vi "main.vi"() -> ()   [LabVIEW 2020]
uses:
  Function/TypeDef/TestFlow.ctl
  <vilib>/Utility/file.llb/Read From Spreadsheet File (string).vi
  <vilib>/Utility/file.llb/Write Delimited Spreadsheet (string).vi
  <vilib>/Utility/file.llb/Read Delimited Spreadsheet (string).vi
panel:
  out "Counter":cluster{"第n筆":u32, "第N輪":u32, "經過時間(ms)":u32}={"第n筆"=1, "第N輪"=1, "經過時間(ms)"=0}
  in  "Test Condition":T1={"每一輪取n筆"=1, "每一輪間隔t時間(sec)"=30.0, "總共取N輪"=1, "開始自動測試"=FALSE} {"總共取N輪" min=1 max=10000; "每一輪間隔t時間(sec)" min=0.01 max=30000.0 format="%_3g"; "每一輪取n筆" min=1 max=10000}
  out "SPR efficiency":dbl
  out "SPR wavelength(nm)":dbl
  in  "結束測試":bool
  in  "OSA Setting":T2={"CENTER(nm)"="850", "SPAN(nm)"="700", "RESOLUTION(nm)"="10", "SAMPLING(point)"="1001", "NEARBY AVG(point)"=50} {"NEARBY AVG(point)" min=0 max=300}
  in  "Tab Control":T3(tab)
  out "P0(air)":cluster{dbl[], dbl[]}(graph)
  out "p test":cluster{dbl[], dbl[]}(graph)
  out "Transmittance":cluster{dbl[], dbl[]}(graph)
  in  "Summarty Folder path":path=path "D:/AQ-6315A RECORD/2012年9月7日/新資料夾"
  in  "疊圖":bool
  out "?":cluster{"appended array":dbl[], dbl[]}[](graph)
  out "?":cluster{"appended array":dbl[], dbl[]}[](graph)
  out "?":path[](array[path])=[path "D:/AQ-6315A RECORD/2012年9月7日/新資料夾/test1-summary.csv", path "D:/AQ-6315A RECORD/2012年9月7日/新資料夾/test2-summary.csv"]
  # "電子系光電實驗室 林鈺城"
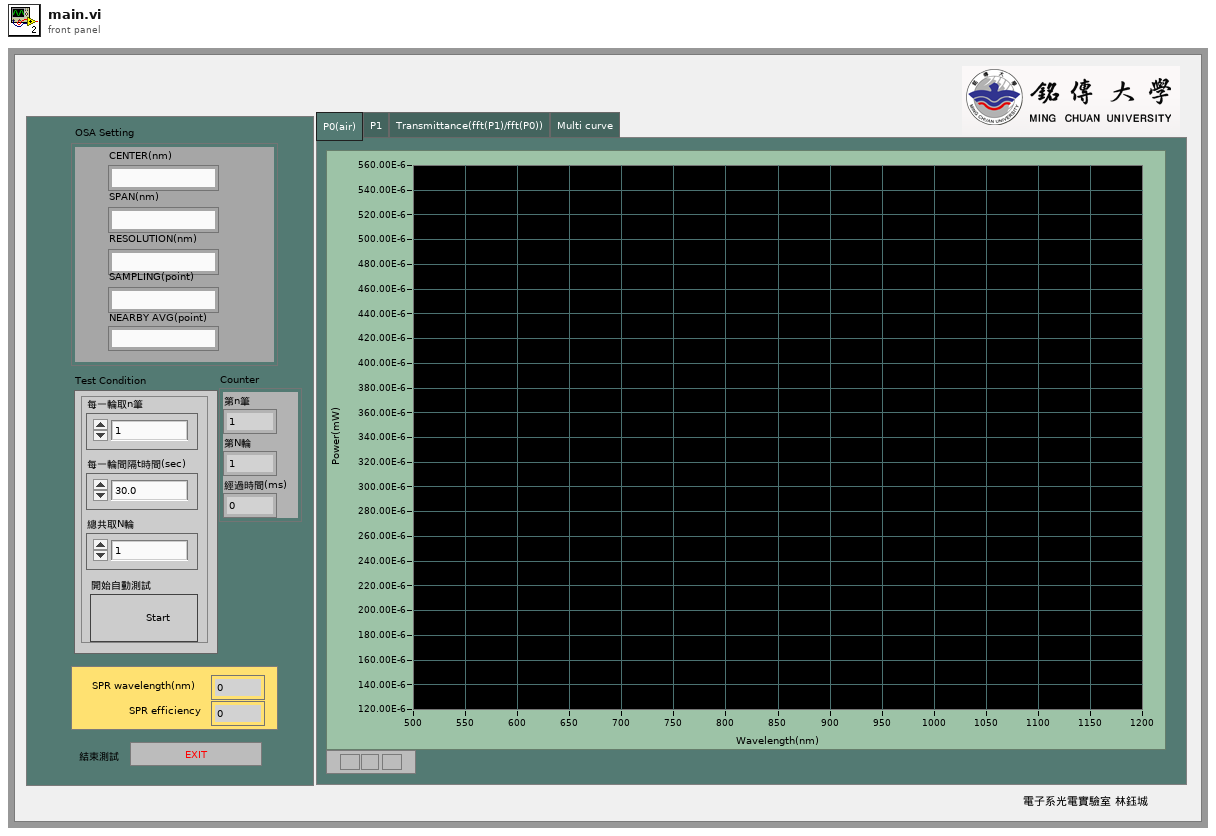
[diagram p1: front panel]
types:
  T1 = cluster{"每一輪取n筆":u32, "每一輪間隔t時間(sec)":dbl, "總共取N輪":u32, "開始自動測試":bool}
  T2 = cluster{"CENTER(nm)":string, "SPAN(nm)":string, "RESOLUTION(nm)":string, "SAMPLING(point)":string, "NEARBY AVG(point)":i32}
  T3 = enum32{"P0(air)", "P1", "Transmittance(fft(P1)/fft(P0))", "Multi curve"}
  T4 = typedef "TestFlow.ctl" = enum16{"Start", "Get P0(air)", "Get P1", "Data process", "Save data", "Continue?", "Finish"}
  T5 = cluster{"P0 Wavelength(nm)":dbl[], "P0 Power(Raw)":dbl[]}
  T6 = cluster{"P1 Wavelength(nm)":dbl[], "P1 Power(Raw)":dbl[]}
  T7 = cluster{"Transmittance":dbl[], "SPR wavelength(nm)":dbl, "SPR efficiency(nm)":dbl, "P0'":dbl[], "P1'":dbl[]}
  T8 = cluster{"P0 Wavelength(nm)":dbl[], "Transmittance":dbl[]}
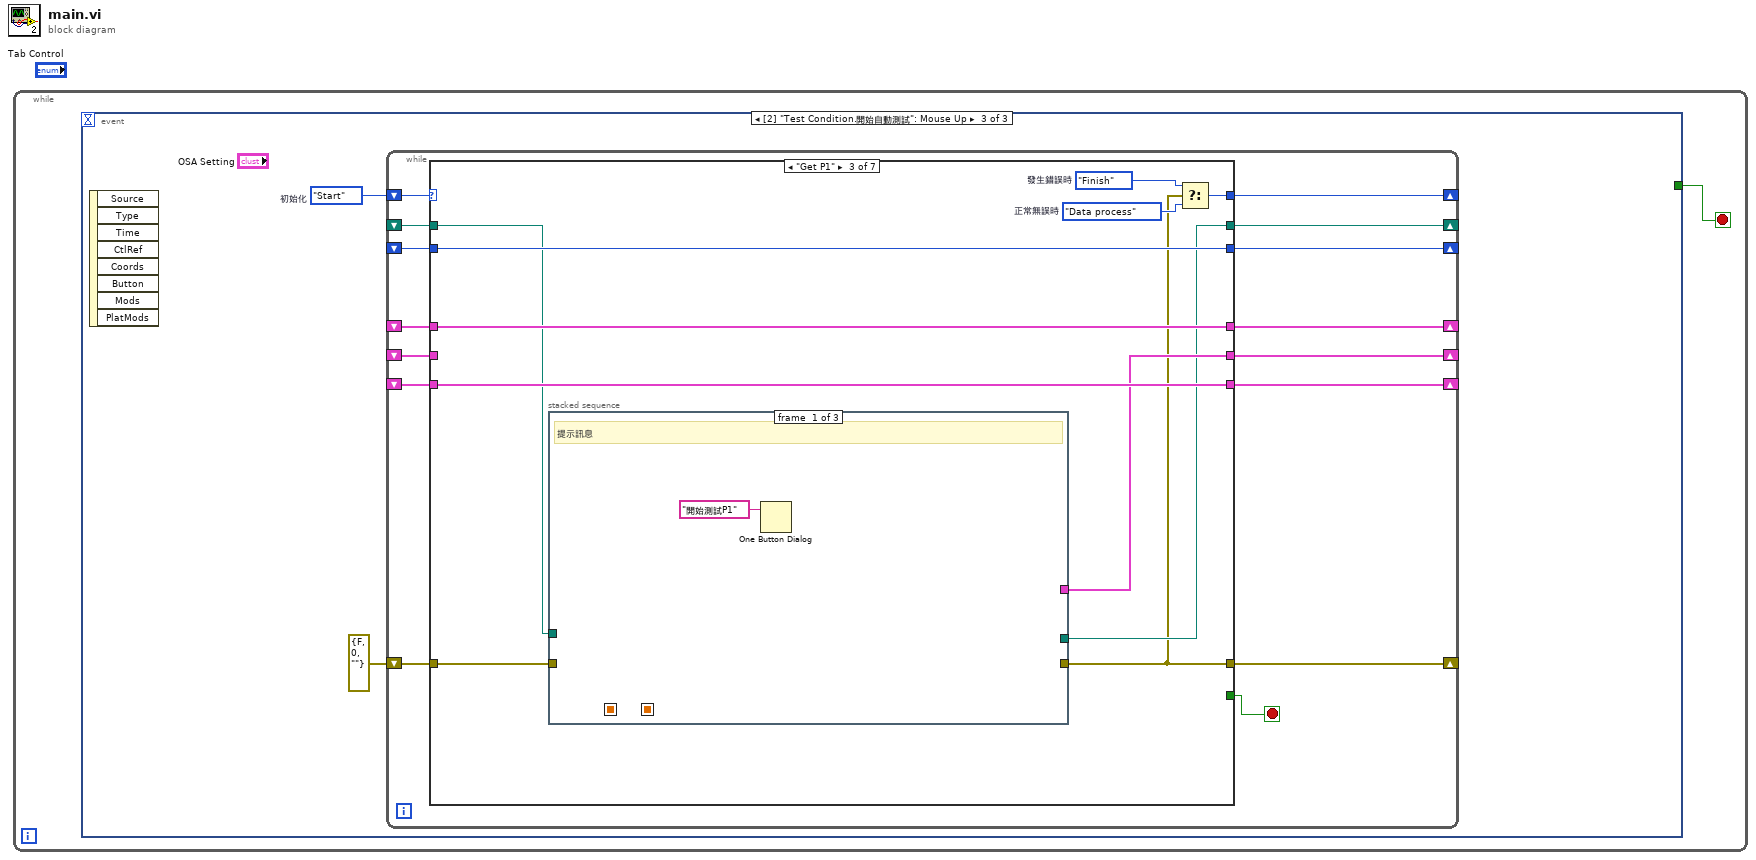
[diagram p0: block diagram]
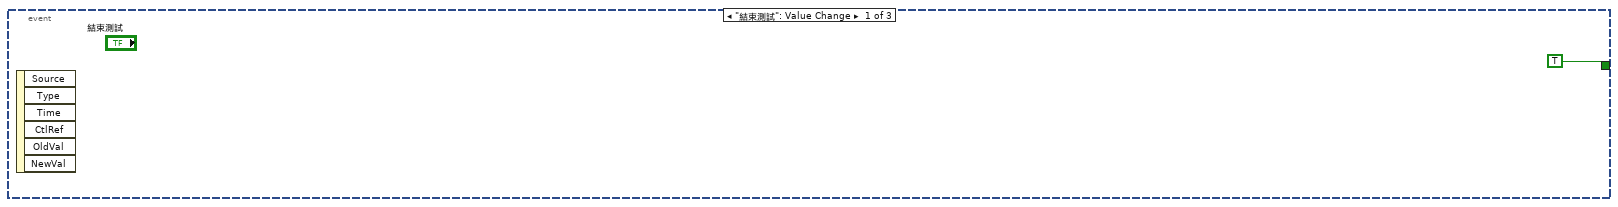
[diagram p2: hidden frame]
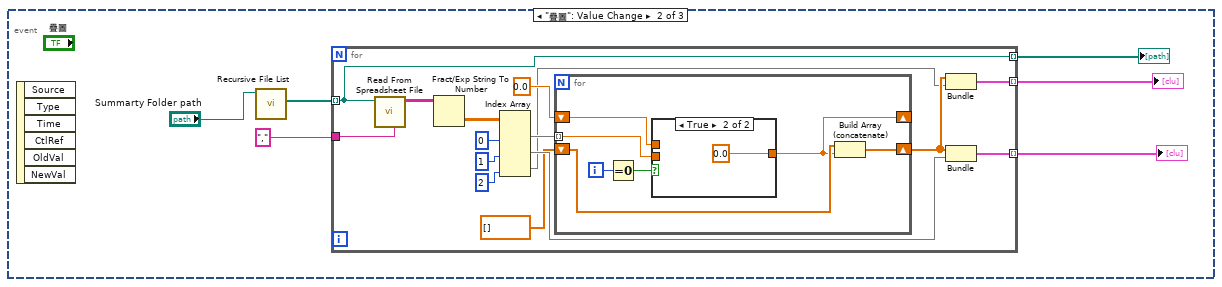
[diagram p3: hidden frame]
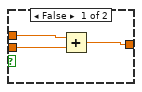
[diagram p4: hidden frame]
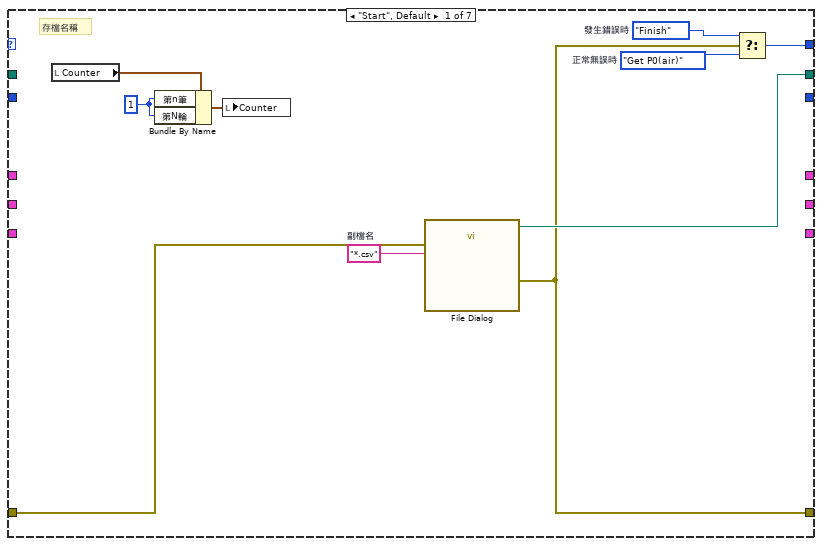
[diagram p5: hidden frame]
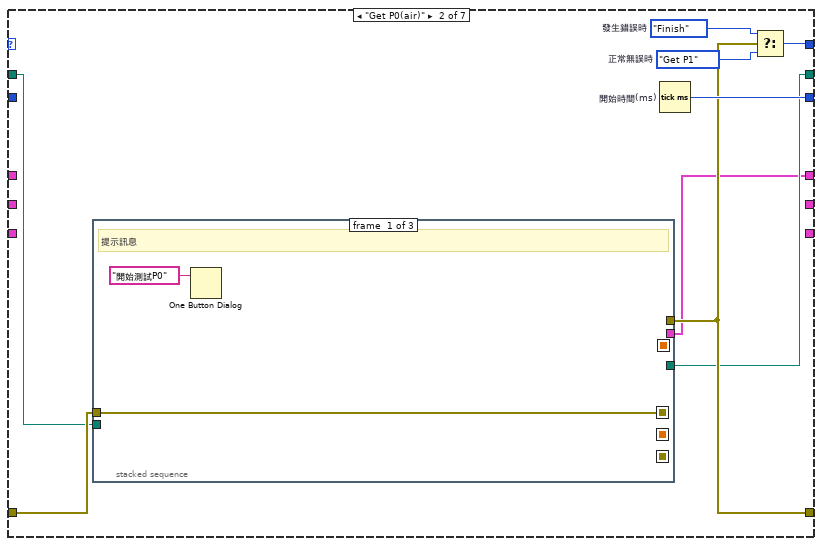
[diagram p6: hidden frame]
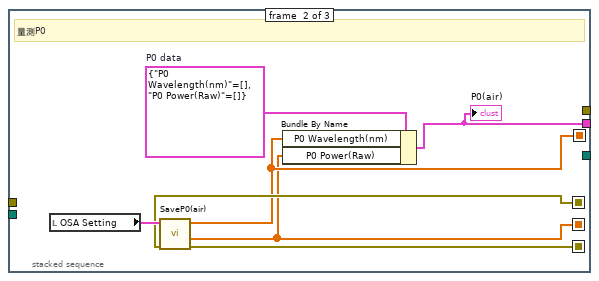
[diagram p7: hidden frame]
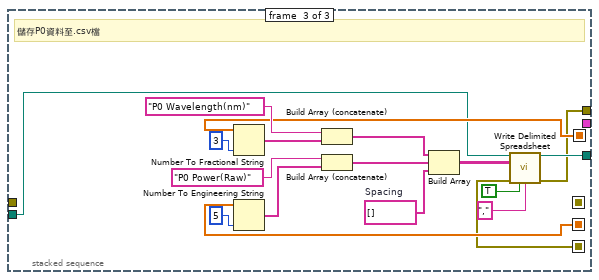
[diagram p8: hidden frame]
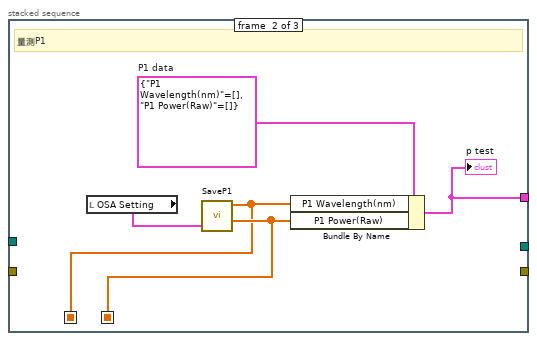
[diagram p9: hidden frame]
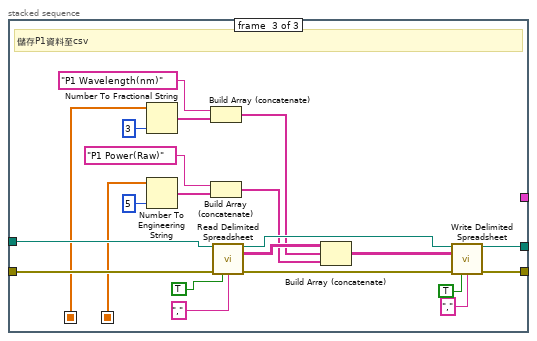
[diagram p10: hidden frame]
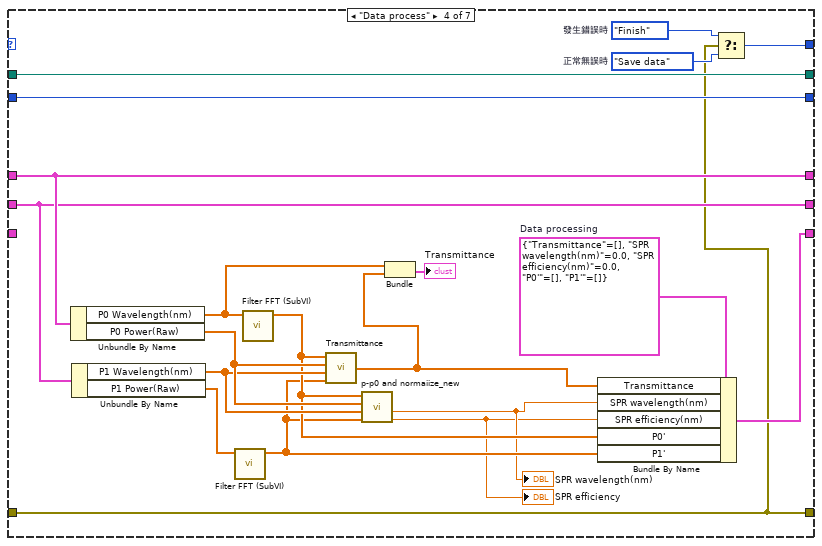
[diagram p11: hidden frame]
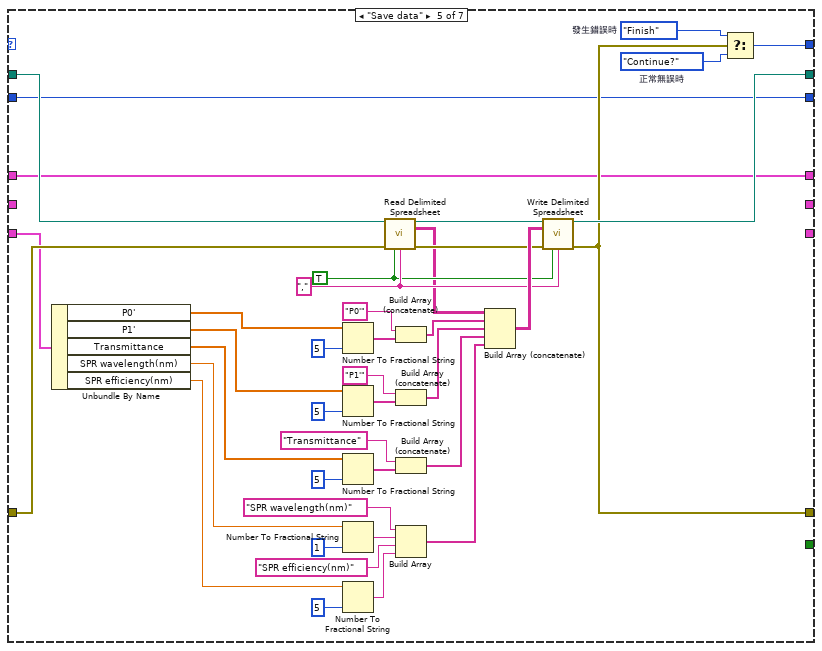
[diagram p12: hidden frame]
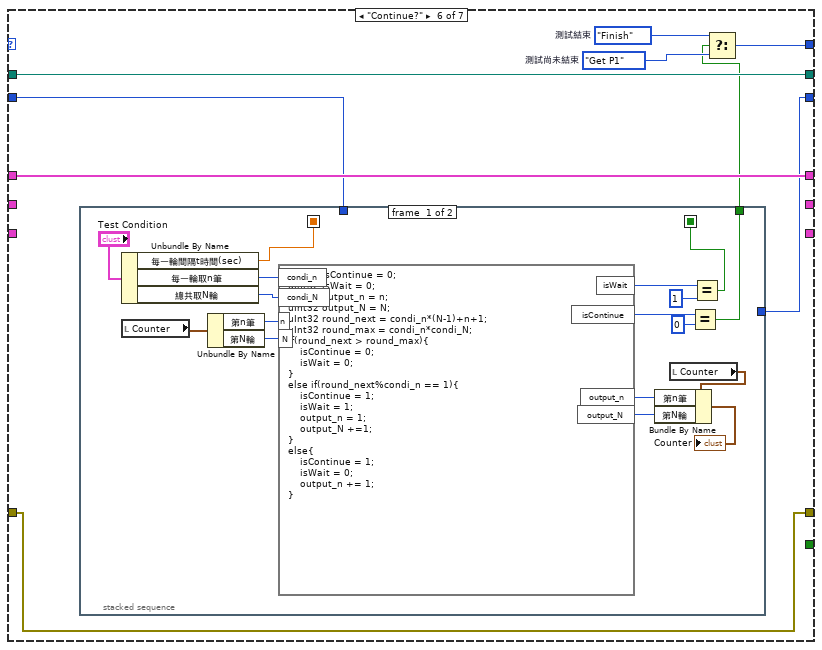
[diagram p13: hidden frame]
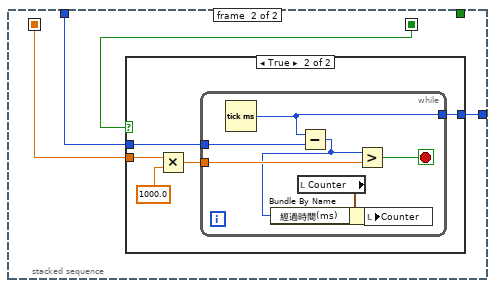
[diagram p14: hidden frame]
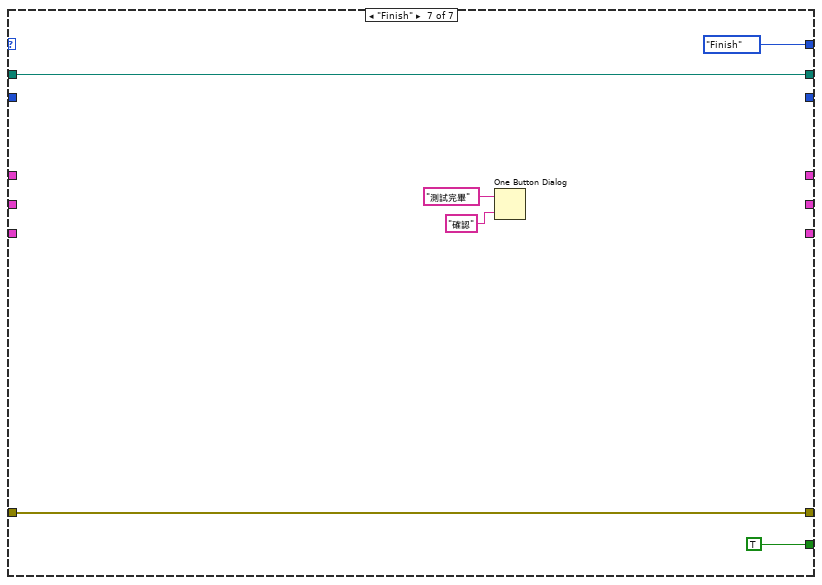
[diagram p16: hidden frame]
diagram:
  n1 = while {
    stop <- w1 stop-if-true
    n2 = event shown="[2] \"Test Condition.開始自動測試\": Mouse Up" {
      selector: _ -> [_ _ _]
      dyn-events: _ -> [_ _ _]
      timeout: _ -> [_ _ _]
      tunnel: [TRUE _ _] -> w1
      event "結束測試": Value Change {
        n3 = event-data() -> ()  [unwired: 7 out]
      }
      event "疊圖": Value Change {
        n4 = event-data() -> ()  [unwired: 7 out]
        n5 = call <vilib>:"Recursive File List.vi"("Folder Path"="Summarty Folder path") -> ("All Files in Dir"=w8:path[])  [unwired: 2 in, 8 out]
        n6 = for {
          tunnel: w8 -> [w9] mode=indexing
          tunnel: "," ("delimiter (\\t)") -> [w20]
          tunnel: [w15] -> w5 mode=indexing
          tunnel: [w12] -> w3 mode=indexing
          tunnel: [w9] -> w4 mode=indexing
          n7 = call-poly <vilib>:"Read From Spreadsheet File.vi"("delimiter (\\t)"=w20, "file path (dialog if empty)"=w9) -> ("all rows"=w19:string[][])  [unwired: 3 in, 6 out]
          n8 = Fract/Exp String To Number(string=w19) -> (number=w18:dbl[][])  [unwired: 4 out]
          n9 = Index Array(array=w18, index (col) #1=0 ("disabled index (col)"), index (col) #2=1 ("index (col)"), index (col) #3=2 ("index (col)")) -> (element #1=w17:dbl[], element #2=w21:dbl[], element #3=w10:dbl[])  [unwired: 3 in]
          n10 = for {
            tunnel: w17 -> [w28] mode=indexing
            shift-right: [w27] -> w13
            shift-left: dbl[] [] ("appended array") -> [w26]
            shift-right: [w24] -> _
            shift-left: 0.0 -> [w25]
            i -> [w30]
            n11 = Equal To 0?(x=w30) -> (x = 0?=w29:bool)
            n12 = case shown="True" w29 {
              tunnel: w28 -> [w33 _]
              tunnel: w25 -> [w32 _]
              tunnel: [w31 0.0 ("String")] -> w24
              frame False {
                n13 = Add(x=w32, y=w33) -> (x+y=w31:dbl)
              }
              frame True {
              }
            }
            n14 = Build Array (concatenate)(w26, w24) -> (w27:dbl[])
          }
          n15 = Bundle("appended array"=w13, w10) -> (w12:cluster{"appended array":dbl[], dbl[]})  [unwired: 1 out]
          n16 = Bundle("appended array"=w13, w21) -> (w15:cluster{"appended array":dbl[], dbl[]})  [unwired: 1 out]
        }
        "?" <- w5
        "?" <- w4
        "?" <- w3
      }
      event "Test Condition.開始自動測試": Mouse Up {
        w36 = TestFlow."Start"  # 初始化
        n17 = event-data() -> ()  [unwired: 9 out]
        n18 = while {
          shift-right: [w47] -> _
          shift-left: w36 -> [w51]
          shift-right: [w50] -> _
          shift-left: _ -> [w45]
          shift-right: [w49] -> _
          shift-left: errorcluster {"status"=FALSE, "code"=0, "source"=""} ("error out") -> [w48]
          shift-right: [w38] -> _
          shift-left: _ -> [w46]
          shift-right: [w40] -> _
          shift-left: _ -> [w44]
          shift-right: [w42] -> _
          shift-left: _ -> [w43]
          shift-right: [w37] -> _
          shift-left: _ -> [w41]
          stop <- w39 stop-if-true
          n19 = case shown="\"Get P1\"" w51 {
            tunnel: [_ _ _ _ _ _ TRUE] -> w39
            tunnel: [w60 w64 w99 w151 w182 w200 w239] -> w50
            tunnel: [w58 w65 w98 w145 w180 w201 w240] -> w49
            tunnel: w48 -> [w59 w70 w100 w145 w188 w201 w240]
            tunnel: [w55 w67 w106 w153 w189 w204 TestFlow."Finish" ("發生錯誤時")] -> w47
            tunnel: [_ w62 w104 w147 w173 w199 _] -> w38
            tunnel: w46 -> [_ _ w104 w147 w173 w199 _]
            tunnel: w45 -> [_ w63 w101 w151 w179 w200 w239]
            tunnel: [_ w66 w105 w152 w172 w196 _] -> w40
            tunnel: w44 -> [_ _ w105 w152 w172 w197 _]
            tunnel: w43 -> [_ _ w103 _ w187 _ _]
            tunnel: [_ _ w103 w148 _ _ _] -> w42
            tunnel: [_ _ w102 w146 _ _ _] -> w37
            tunnel: w41 -> [_ _ _ w146 _ _ _]
            frame "Start", Default {
              w53 = u32 1 ("第n筆")
              w57 = TestFlow."Get P0(air)"  # 正常無誤時
              w56 = TestFlow."Finish"  # 發生錯誤時
              w61 = "*.csv"  # 副檔名
              # "存檔名稱"
              n20 = local read "Counter"() -> (w54:cluster{"第n筆":u32, "第N輪":u32, "經過時間(ms)":u32})
              n21 = Bundle By Name(cluster=w54, "第n筆"=w53, "第N輪"=w53) -> (w52:cluster{"第n筆":u32, "第N輪":u32, "經過時間(ms)":u32})
              n22 = local write "Counter"(w52) -> ()
              n23 = call "File Dialog"("error in"=w59, "pattern (all files)"=w61) -> ("selected path"=w60:path, "error out"=w58:errorcluster)  [unwired: 10 in, 2 out]
              n24 = Select(t=w56, s=w58, f=w57) -> (s? t:f=w55:T4)
            }
            frame "Get P0(air)" {
              w68 = TestFlow."Get P1"  # 正常無誤時
              w69 = TestFlow."Finish"  # 發生錯誤時
              n25 = stacked-sequence {
                seq-local: [w71 _ _] -> [_ w77 _]
                seq-local: [_ w76 _] -> [_ _ w92]
                seq-local: [_ w75 _] -> [_ _ w87]
                seq-local: [_ w78 _] -> [_ _ w85]
                tunnel: w70 -> [w71 _ _]
                tunnel: w63 -> [_ _ w81]
                tunnel: [_ _ w86] -> w64
                tunnel: [_ _ w80] -> w65
                tunnel: [_ w73 _] -> w62
                frame #0 {
                  # "提示訊息"
                  n26 = One Button Dialog(message="開始測試P0") -> ()  [unwired: 1 in, 1 out]
                }
                frame #1 {
                  w74 = T5 {"P0 Wavelength(nm)"=[], "P0 Power(Raw)"=[]}  # P0 data
                  # "量測P0"
                  n27 = local read "OSA Setting"() -> (w79:T2)
                  n28 = call "SaveP0(air).vi"("error in (no error)"=w77, "OSA Setting"=w79) -> ("error out"=w78:errorcluster, "Power"=w75:dbl[], "Wavelength"=w76:dbl[])  [unwired: 6 in]
                  n29 = Bundle By Name(cluster=w74, "P0 Wavelength(nm)"=w76, "P0 Power(Raw)"=w75) -> (w73:T5)
                  "P0(air)" <- w73
                }
                frame #2 {
                  w82 = string[] []  # Spacing
                  # "儲存P0資料至.csv檔"
                  n30 = Number To Fractional String(number=w92, precision (6)=i16 3) -> (F-format string=w95:string[])  [unwired: 2 in]
                  n31 = Number To Engineering String(2:i16 5 ("precision (6)"), 4:w87) -> (0:w89:string[])  [unwired: 2 in]
                  n32 = Build Array (concatenate)("P0 Wavelength(nm)", w95) -> (w97:string[])
                  n33 = Build Array (concatenate)("P0 Power(Raw)", w89) -> (w88:string[])
                  n34 = Build Array(w97, w88, w82) -> (w96:string[][])
                  n35 = call-poly <vilib>:"Write Delimited Spreadsheet.vi"("file path (dialog if empty)"=w81, "2D data"=w96, "error in (no error)"=w85, "transpose? (no:F)"=TRUE, "delimiter (\\t)"="," ("delimiter (\\t)")) -> ("new file path (Not A Path if cancelled)"=w86:path, "error out"=w80:errorcluster)  [unwired: 9 in]
                }
              }
              n36 = Tick Count (ms) "開始時間(ms)"() -> (millisecond timer value=w66:u32)
              n37 = Select(t=w69, s=w65, f=w68) -> (s? t:f=w67:T4)
            }
            frame "Get P1" {
              w107 = TestFlow."Data process"  # 正常無誤時
              w108 = TestFlow."Finish"  # 發生錯誤時
              n38 = stacked-sequence {
                seq-local: [_ w112 _] -> [_ _ w117]
                seq-local: [_ w111 _] -> [_ _ w118]
                tunnel: [_ w110 _] -> w102
                tunnel: w101 -> [_ _ w127]
                tunnel: w100 -> [_ _ w126]
                tunnel: [_ _ w120] -> w99
                tunnel: [_ _ w119] -> w98
                frame #0 {
                  # "提示訊息"
                  n39 = One Button Dialog(message="開始測試P1") -> ()  [unwired: 1 in, 1 out]
                }
                frame #1 {
                  w113 = T6 {"P1 Wavelength(nm)"=[], "P1 Power(Raw)"=[]}  # P1 data
                  # "量測P1"
                  n40 = local read "OSA Setting"() -> (w114:T2)
                  n41 = call "SaveP1.vi"("OSA Setting"=w114) -> ("Power"=w112:dbl[], "Wavelength"=w111:dbl[])  [unwired: 9 in]
                  n42 = Bundle By Name(cluster=w113, "P1 Wavelength(nm)"=w111, "P1 Power(Raw)"=w112) -> (w110:T6)
                  "p test" <- w110
                }
                frame #2 {
                  # "儲存P1資料至csv"
                  n43 = Number To Fractional String(number=w118, precision (6)=i16 3) -> (F-format string=w132:string[])  [unwired: 2 in]
                  n44 = Number To Engineering String(2:i16 5 ("precision (6)"), 4:w117) -> (0:w131:string[])  [unwired: 2 in]
                  n45 = Build Array (concatenate)("P1 Wavelength(nm)", w132) -> (w133:string[])
                  n46 = Build Array (concatenate)("P1 Power(Raw)", w131) -> (w130:string[])
                  n47 = call-poly <vilib>:"Read Delimited Spreadsheet.vi"("file path (dialog if empty)"=w127, "error in (no error)"=w126, "transpose? (F)"=TRUE ("transpose? (no:F)"), "delimiter (\\t)"="," ("delimiter (\\t)")) -> ("new file path (Not A Path if cancelled)"=w134:path, "all rows"=w136:string[][], "error out"=w135:errorcluster)  [unwired: 6 in, 3 out]
                  n48 = Build Array (concatenate)(w136, w133, w130) -> (w129:string[][])
                  n49 = call-poly <vilib>:"Write Delimited Spreadsheet.vi"("file path (dialog if empty)"=w134, "2D data"=w129, "error in (no error)"=w135, "transpose? (no:F)"=TRUE, "delimiter (\\t)"="," ("delimiter (\\t)")) -> ("new file path (Not A Path if cancelled)"=w120:path, "error out"=w119:errorcluster)  [unwired: 9 in]
                }
              }
              n50 = Select(t=w108, s=w98, f=w107) -> (s? t:f=w106:T4)
            }
            frame "Data process" {
              w149 = T7 {"Transmittance"=[], "SPR wavelength(nm)"=0.0, "SPR efficiency(nm)"=0.0, "P0'"=[], "P1'"=[]}  # Data processing
              w154 = TestFlow."Save data"  # 正常無誤時
              w155 = TestFlow."Finish"  # 發生錯誤時
              n51 = Unbundle By Name(w147) -> ("P0 Wavelength(nm)"=w139:dbl[], "P0 Power(Raw)"=w156:dbl[])
              n52 = Unbundle By Name(w146) -> ("P1 Wavelength(nm)"=w150:dbl[], "P1 Power(Raw)"=w144:dbl[])
              n53 = call "Filter FFT (SubVI).vi"("Input"=w144) -> ("Output"=w142:dbl[])  [unwired: 10 in]
              n54 = call "Filter FFT (SubVI).vi"("Input"=w139) -> ("Output"=w143:dbl[])  [unwired: 10 in]
              n55 = call "Transmittance.vi"("P1 Power"=w142, "P1 Wavelength"=w150, "P0 Power"=w156, "P0 Wavelength"=w143) -> ("Transmittance"=w137:dbl[])
              n56 = call "p-p0 and normaiize_new.vi"("P1 power"=w142, "P1 wavelength"=w150, "P0 power"=w156, "P0 wavelength"=w143) -> ("SPR efficiency"=w140:dbl, "SPR wave length(nm)"=w141:dbl)  [unwired: 1 in, 1 out]
              "SPR wavelength(nm)" <- w141
              "SPR efficiency" <- w140
              n57 = Bundle("P0 Wavelength(nm)"=w139, "Transmittance"=w137) -> (→"Transmittance":T8)  [unwired: 1 in]
              n58 = Bundle By Name(cluster=w149, "Transmittance"=w137, "SPR wavelength(nm)"=w141, "SPR efficiency(nm)"=w140, "P0'"=w143, "P1'"=w142) -> (w148:T7)
              n59 = Select(t=w155, s=w145, f=w154) -> (s? t:f=w153:T4)
            }
            frame "Save data" {
              w190 = TestFlow."Continue?"  # 正常無誤時
              w191 = TestFlow."Finish"  # 發生錯誤時
              w176 = TRUE ("transpose? (no:F)")
              w177 = "," ("delimiter (\\t)")
              n60 = Unbundle By Name(w187) -> ("P0'"=w162:dbl[], "P1'"=w161:dbl[], "Transmittance"=w163:dbl[], "SPR wavelength(nm)"=w170:dbl, "SPR efficiency(nm)"=w169:dbl)
              n61 = Number To Fractional String(number=w162, precision (6)=i16 5) -> (F-format string=w168:string[])  [unwired: 2 in]
              n62 = Number To Fractional String(number=w161, precision (6)=i16 5) -> (F-format string=w165:string[])  [unwired: 2 in]
              n63 = Number To Fractional String(number=w163, precision (6)=i16 5) -> (F-format string=w184:string[])  [unwired: 2 in]
              n64 = Number To Fractional String(number=w170, precision (6)=i16 1) -> (F-format string=w195:string)  [unwired: 2 in]
              n65 = Number To Fractional String(number=w169, precision (6)=i16 5) -> (F-format string=w174:string)  [unwired: 2 in]
              n66 = call-poly <vilib>:"Read Delimited Spreadsheet.vi"("file path (dialog if empty)"=w179, "transpose? (F)"=w176, "delimiter (\\t)"=w177) -> ("new file path (Not A Path if cancelled)"=w178:path, "all rows"=w159:string[][])  [unwired: 7 in, 4 out]
              n67 = Build Array (concatenate)("P0'", w168) -> (w157:string[])
              n68 = Build Array (concatenate)("P1'", w165) -> (w158:string[])
              n69 = Build Array (concatenate)("Transmittance", w184) -> (w183:string[])
              n70 = Build Array("SPR wavelength(nm)", w195, "SPR efficiency(nm)", w174) -> (w171:string[])
              n71 = Build Array (concatenate)(w159, w157, w158, w183, w171) -> (w194:string[][])
              n72 = call-poly <vilib>:"Write Delimited Spreadsheet.vi"("file path (dialog if empty)"=w178, "2D data"=w194, "error in (no error)"=w188, "transpose? (no:F)"=w176, "delimiter (\\t)"=w177) -> ("new file path (Not A Path if cancelled)"=w182:path, "error out"=w180:errorcluster)  [unwired: 9 in]
              n73 = Select(t=w191, s=w180, f=w190) -> (s? t:f=w189:T4)
            }
            frame "Continue?" {
              w202 = TestFlow."Finish"  # 測試結束
              w203 = TestFlow."Get P1"  # 測試尚未結束
              n74 = stacked-sequence {
                seq-local: [w206 _] -> [_ w223]
                seq-local: [w205 _] -> [_ w222]
                tunnel: [w212 _] -> w198
                tunnel: w197 -> [_ w225]
                tunnel: [_ w224] -> w196
                frame #0 {
                  n75 = Unbundle By Name("Test Condition") -> ("每一輪間隔t時間(sec)"=w205:dbl, "每一輪取n筆"=w211:u32, "總共取N輪"=w210:u32)
                  n76 = local read "Counter"() -> (w216:cluster{"第n筆":u32, "第N輪":u32, "經過時間(ms)":u32})
                  n77 = Unbundle By Name(w216) -> ("第n筆"=w209:u32, "第N輪"=w208:u32)
                  n78 = formula code="uInt32 isContinue = 0;\nuInt32 isWait = 0;\nuInt32 output_n = n;\nuInt32 output_N = N;\nuInt32 round_next = condi_n*(N-1)+n+1;\nuInt32 round_max = condi_n*condi_N;\nif(round_next > round_max){\n    isContinue = 0;\n    isWait = 0;\n}\nelse if(round_next%condi_n == 1){\n    isContinue = 1;\n    isWait = 1;\n    output_n = 1;\n    output_N +=1;\n}\nelse{\n    isContinue = 1;\n    isWait = 0;\n    output_n += 1;\n}"("n"=w209, "N"=w208, "condi_n"=w211, "condi_N"=w210) -> ("isContinue"=w217:u32, "isWait"=w218:u32, "output_n"=w220:u32, "output_N"=w207:u32)
                  n79 = local read "Counter"() -> (w219:cluster{"第n筆":u32, "第N輪":u32, "經過時間(ms)":u32})
                  n80 = Bundle By Name(cluster=w219, "第n筆"=w220, "第N輪"=w207) -> (→"Counter":cluster{"第n筆":u32, "第N輪":u32, "經過時間(ms)":u32})
                  n81 = Equal?(x=w217, y=u32 0) -> (x = y?=w212:bool)
                  n82 = Equal?(x=w218, y=u32 1) -> (x = y?=w206:bool)
                }
                frame #1 {
                  n83 = case shown="True" w223 {
                    tunnel: w222 -> [_ w231]
                    tunnel: w225 -> [w226 w229]
                    tunnel: [w226 w227] -> w224
                    frame False {
                    }
                    frame True {
                      n84 = Multiply(x=w231, y=1000.0) -> (x*y=w228:dbl)
                      n85 = while {
                        tunnel: w229 -> [w238]
                        tunnel: w228 -> [w237]
                        tunnel: [w235] -> w227
                        stop <- w236 stop-if-true
                        n86 = Tick Count (ms)() -> (millisecond timer value=w235:u32)
                        n87 = local read "Counter"() -> (w233:cluster{"第n筆":u32, "第N輪":u32, "經過時間(ms)":u32})
                        n88 = Subtract(x=w235, y=w238) -> (x-y=w232:u32)
                        n89 = Bundle By Name(cluster=w233, "經過時間(ms)"=w232) -> (w234:cluster{"第n筆":u32, "第N輪":u32, "經過時間(ms)":u32})
                        n90 = Greater?(x=w232, y=w237) -> (0:w236:bool)
                        n91 = local write "Counter"(w234) -> ()
                      }
                    }
                  }
                }
              }
              n92 = Select(t=w202, s=w198, f=w203) -> (s? t:f=w204:T4)
            }
            frame "Finish" {
              n93 = One Button Dialog(message="測試完畢", button name ("OK")="確認") -> ()  [unwired: 1 out]
            }
          }
        }
      }
    }
  }
